vi "read.vi"(9 "file path (dialog if empty)":path) -> (2 "Array":T2(array[cluster]))   [LabVIEW 2016]
uses:
  <vilib>/Utility/file.llb/Read Delimited Spreadsheet (DBL).vi
panel:
  out "draw point Cluster":T1
  out "data num":i32
  # "檔案位置"
  # "資料陣列輸出"
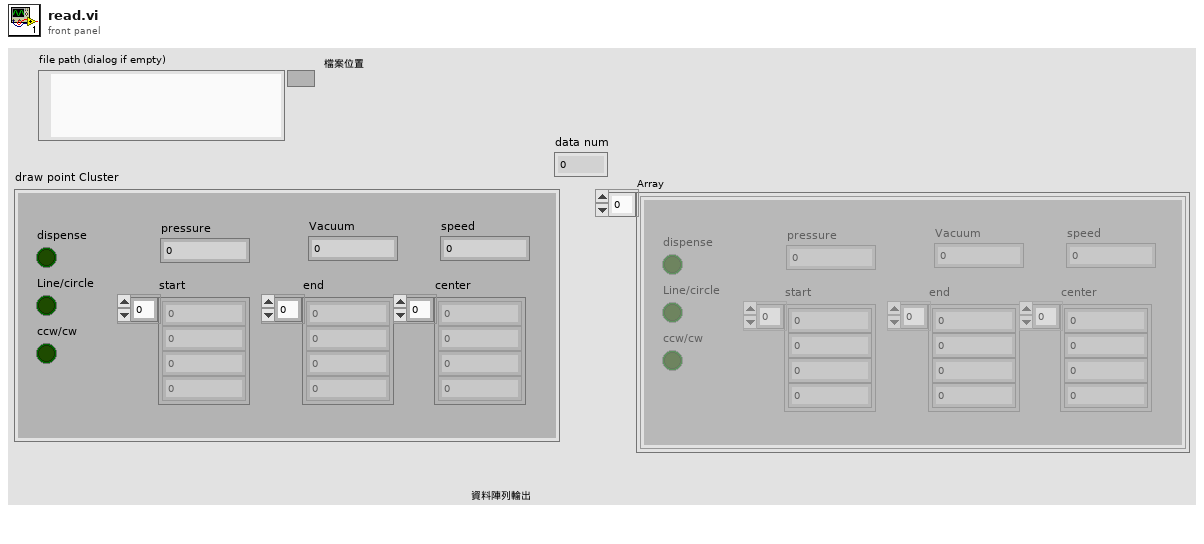
[diagram p1: front panel]
types:
  T1 = cluster{"dispense":bool, "Line/circle":bool, "ccw/cw":bool, "pressure":dbl, "speed":dbl, "start":dbl[], "end":dbl[], "center":dbl[], "Vacuum":dbl}
  T2 = cluster{"dispense":bool, "Line/circle":bool, "ccw/cw":bool, "pressure":dbl, "speed":dbl, "start":dbl[], "end":dbl[], "center":dbl[], "Vacuum":dbl}[]
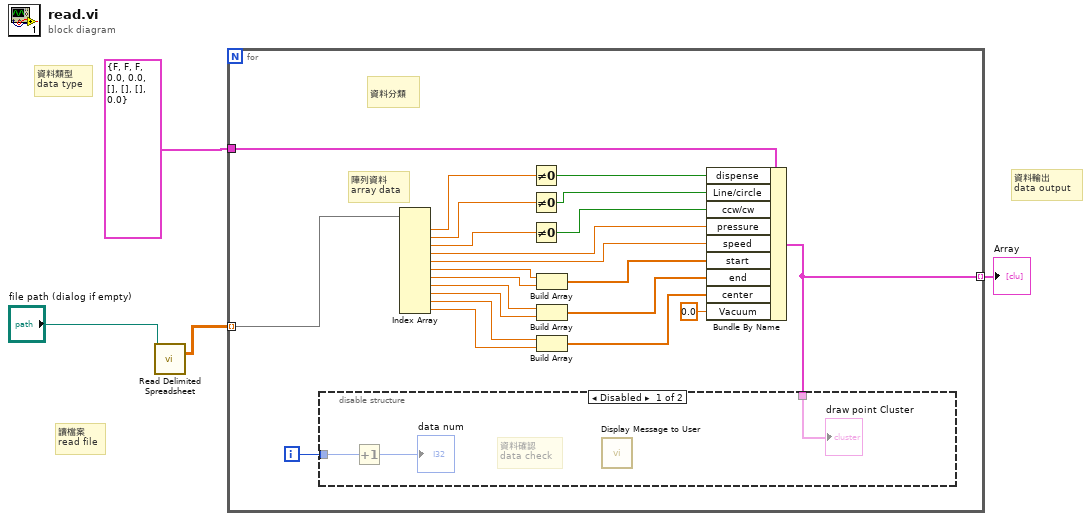
[diagram p0: block diagram]
diagram:
  # "資料類型\ndata type"
  # "資料輸出\ndata output"
  # "讀檔案\nread file"
  n1 = call-poly <vilib>:"Read Delimited Spreadsheet.vi"("file path (dialog if empty)"="file path (dialog if empty)") -> ("all rows"=w3:dbl[][])  [unwired: 9 in, 5 out]
  n2 = for {
    tunnel: T1 {"dispense"=FALSE, "Line/circle"=FALSE, "ccw/cw"=FALSE, "pressure"=0.0, "speed"=0.0, "start"=[], "end"=[], "center"=[], "Vacuum"=0.0} ("draw point Cluster") -> [w25]
    tunnel: w3 -> [w26] mode=indexing
    tunnel: [w7] -> w2 mode=indexing
    i -> [w6]
    # "資料分類"
    # "陣列資料\narray data"
    n3 = Index Array(array=w26) -> (element #1=w24:dbl, element #2=w20:dbl, element #3=w19:dbl, element #4=w18:dbl, element #5=w17:dbl, element #6=w16:dbl, element #7=w15:dbl, element #8=w13:dbl, element #9=w12:dbl, element #10=w10:dbl, element #11=w9:dbl)  [unwired: 11 in]
    n4 = Not Equal To 0?(x=w24) -> (x != 0?=w23:bool)
    n5 = Not Equal To 0?(x=w20) -> (x != 0?=w22:bool)
    n6 = Not Equal To 0?(x=w19) -> (x != 0?=w21:bool)
    n7 = Build Array(w16, w15) -> (w14:dbl[])
    n8 = Build Array(w13, w12) -> (w11:dbl[])
    n9 = Build Array(w10, w9) -> (w8:dbl[])
    n10 = Bundle By Name(cluster=w25, "dispense"=w23, "Line/circle"=w22, "ccw/cw"=w21, "pressure"=w18, "speed"=w17, "start"=w14, "end"=w11, "center"=w8, "Vacuum"=0.0) -> (w7:T1)
    n11 = disable-structure shown="Disabled" {
      disable-tunnel: w7 -> [w27 _]
      disable-tunnel: w6 -> [w29 _]
      frame Disabled {
        # "資料確認\ndata check"
        n12 = Increment(x=w29) -> (x+1=→"data num":i32)
        n13 = call "Display Message to User"() -> ()  [unwired: 10 in, 2 out]
        "draw point Cluster" <- w27
      }
      frame Enabled {
      }
    }
  }
  "Array" <- w2
